vi "test_Outgoing1 Waveforms.vi"(8 "error in (no error)":errorcluster, 11 "DMA Channels Basic Testing in":refnum<class "DMA Channels Interleaved Testing.lvclass">) -> (0 "error out":errorcluster, 3 "DMA Channels Basic Testing out":refnum<class "DMA Channels Interleaved Testing.lvclass">)   [LabVIEW 2019, in "DMA Channels Interleaved Testing.lvclass"]
uses:
  DMA Channels Interleaved Testing.lvclass
panel:
  out "Waveform 2":waveform(dbl)(graph)
  out "Waveform 1":waveform(dbl)(graph)
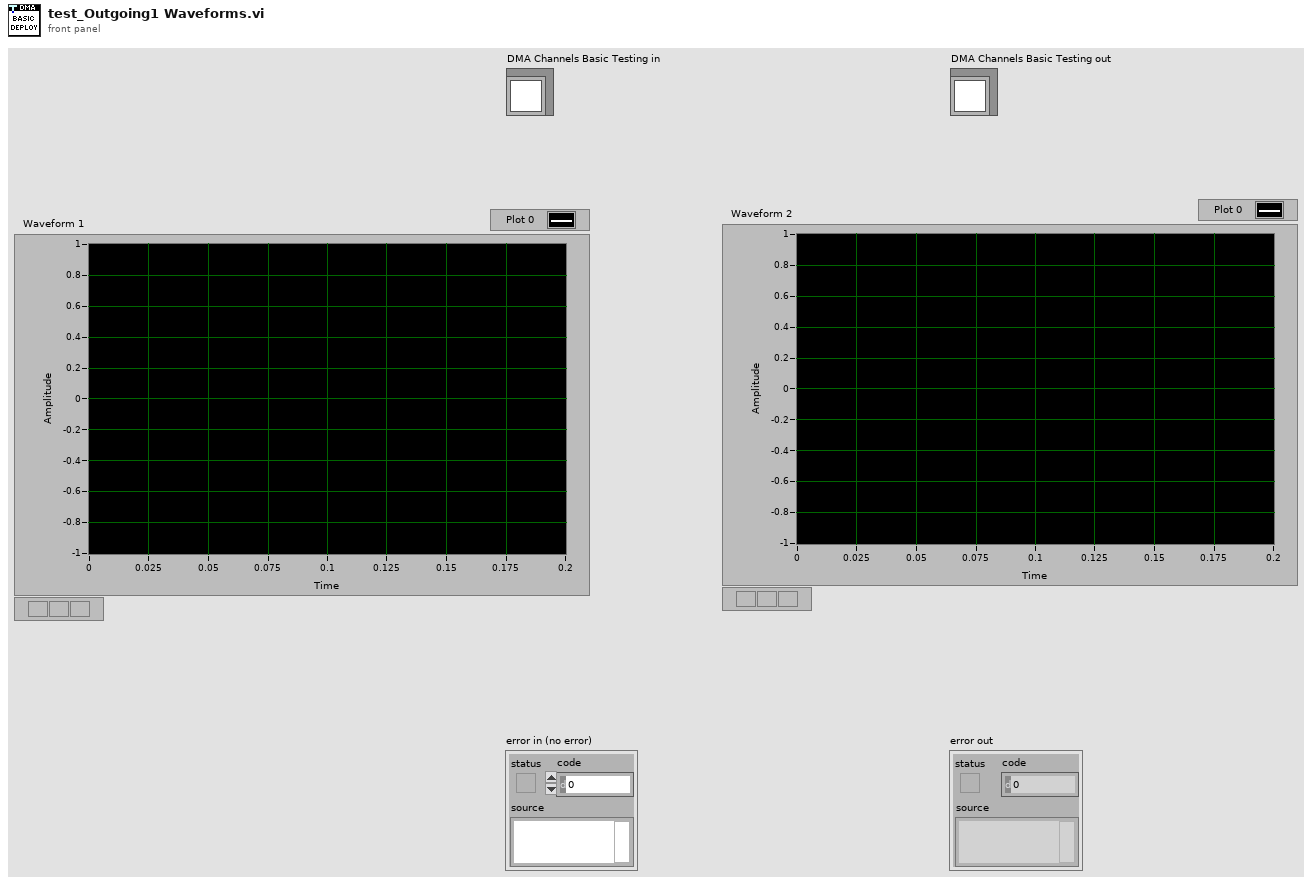
[diagram p1: front panel]
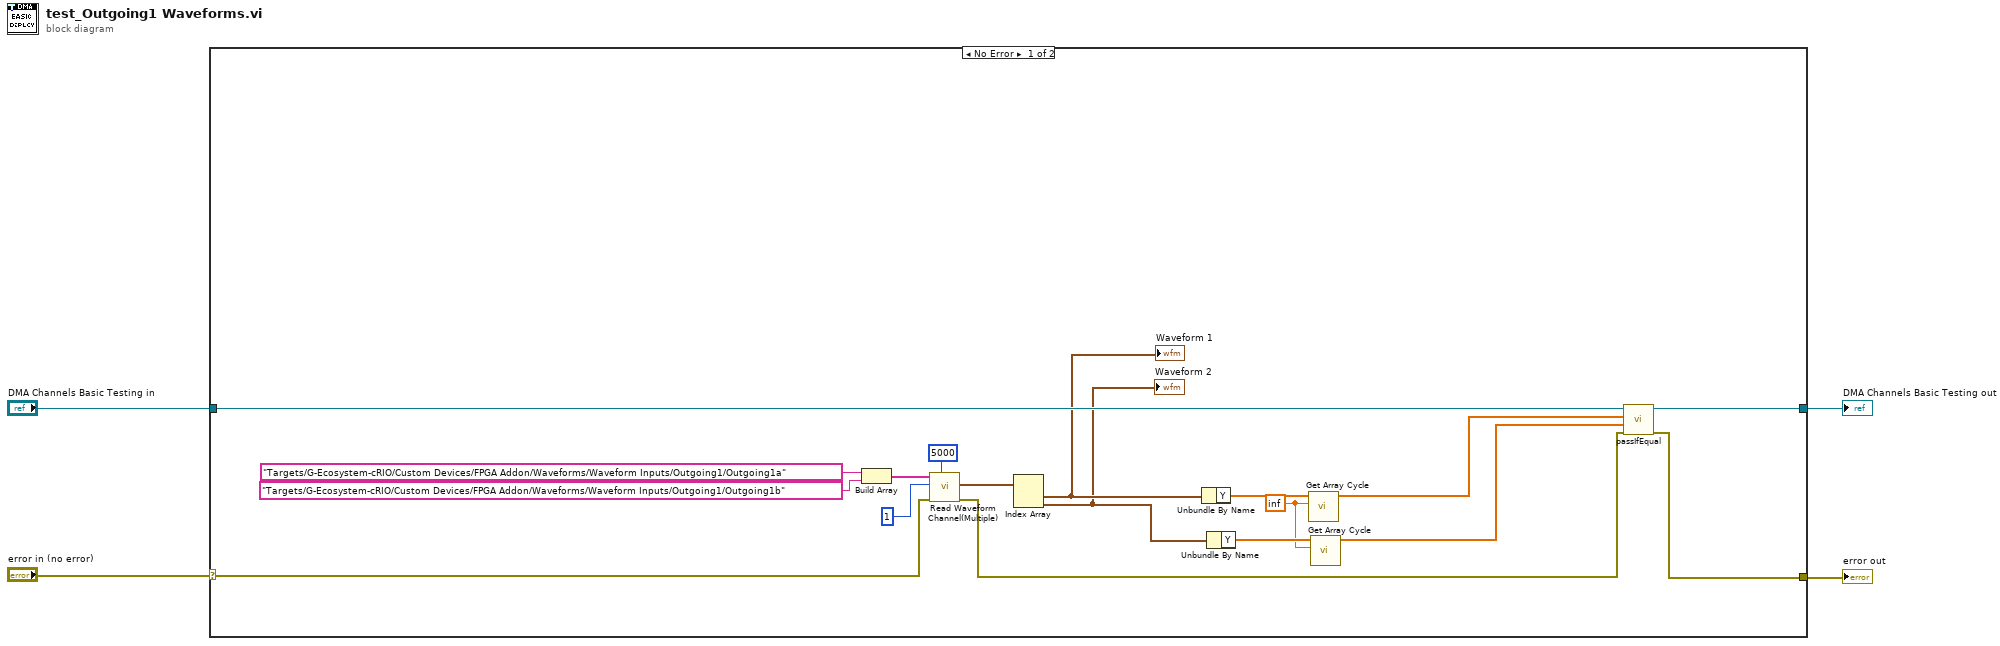
[diagram p0: block diagram]
diagram:
  n1 = case shown="No Error" "error in (no error)" {
    selector: "error in (no error)" -> [w15 w23]
    tunnel: "DMA Channels Basic Testing in" -> [w22 w24]
    tunnel: [w20 w24] -> w1
    tunnel: [w21 w23] -> w3
    frame No Error {
      w9 = inf ("Marker")
      n2 = Build Array("Targets/G-Ecosystem-cRIO/Custom Devices/FPGA Addon/Waveforms/Waveform Inputs/Outgoing1/Outgoing1a" ("waveform path"), "Targets/G-Ecosystem-cRIO/Custom Devices/FPGA Addon/Waveforms/Waveform Inputs/Outgoing1/Outgoing1b" ("waveform path")) -> (w17:string[])
      n3 = call "Read Waveform Channel(Multiple).vi"("Timeout"=5000, "error in (no error)"=w15, "Number of Reads"=1, "Waveform Paths in"=w17) -> ("error out"=w13:errorcluster, "Waveform Data"=w16:waveform(dbl)[])  [unwired: 5 in, 1 out]
      n4 = Index Array(array=w16) -> (element #1=w6:waveform(dbl), element #2=w5:waveform(dbl))  [unwired: 2 in]
      "Waveform 1" <- w6
      "Waveform 2" <- w5
      n5 = Unbundle By Name(w6) -> ("Y"=w11:dbl[])
      n6 = Unbundle By Name(w5) -> ("Y"=w10:dbl[])
      n7 = call "Get Array Cycle.vi"("Marker"=w9, "Array Samples"=w11) -> ("Array"=w8:dbl[])  [unwired: 8 in, 1 out]
      n8 = call "Get Array Cycle.vi"("Marker"=w9, "Array Samples"=w10) -> ("Array"=w7:dbl[])  [unwired: 8 in, 1 out]
      n9 = call-dynamic "passIfEqual.vi"("error in (no error)"=w13, "y"=w7, "x"=w8, "TestCase in"=w22) -> ("error out"=w21:errorcluster, "TestCase out"=w20:refnum<class "DMA Channels Interleaved Testing.lvclass">)  [unwired: 6 in]
    }
    frame Error {
    }
  }
  "error out" <- w3
  "DMA Channels Basic Testing out" <- w1
